vi "task3_BINARY2DEC_CONVERTER.vi"() -> ()   [LabVIEW 2017]
panel:
  out "display":dbl
  in  "2^0":bool
  in  "2^1":bool
  in  "2^2":bool
  in  "2^3":bool
  in  "2^4":bool
  in  "2^5":bool
  in  "2^6":bool
  in  "2^7":bool
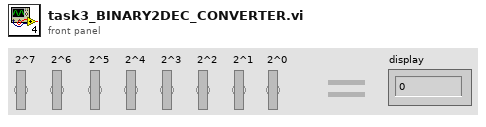
[diagram p1: front panel]
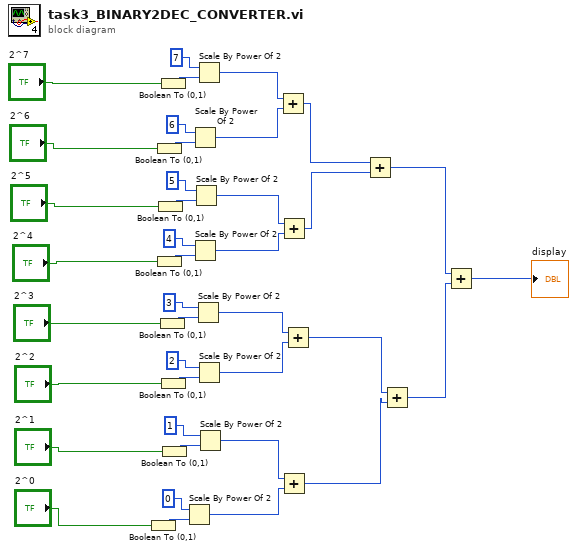
[diagram p0: block diagram]
diagram:
  n1 = Boolean To (0,1)(Boolean="2^0") -> (0, 1=w39:i16)
  n2 = Boolean To (0,1)(Boolean="2^6") -> (0, 1=w33:i16)
  n3 = Boolean To (0,1)(Boolean="2^4") -> (0, 1=w35:i16)
  n4 = Boolean To (0,1)(Boolean="2^5") -> (0, 1=w34:i16)
  n5 = Boolean To (0,1)(Boolean="2^3") -> (0, 1=w36:i16)
  n6 = Boolean To (0,1)(Boolean="2^7") -> (0, 1=w32:i16)
  n7 = Boolean To (0,1)(Boolean="2^2") -> (0, 1=w37:i16)
  n8 = Boolean To (0,1)(Boolean="2^1") -> (0, 1=w38:i16)
  n9 = Scale By Power Of 2(n=0, x=w39) -> (x*2^n=w16:i16)
  n10 = Scale By Power Of 2(n=6, x=w33) -> (x*2^n=w22:i16)
  n11 = Scale By Power Of 2(n=4, x=w35) -> (x*2^n=w20:i16)
  n12 = Scale By Power Of 2(n=5, x=w34) -> (x*2^n=w21:i16)
  n13 = Scale By Power Of 2(n=3, x=w36) -> (x*2^n=w19:i16)
  n14 = Scale By Power Of 2(n=7, x=w32) -> (x*2^n=w23:i16)
  n15 = Scale By Power Of 2(n=2, x=w37) -> (x*2^n=w18:i16)
  n16 = Scale By Power Of 2(n=1, x=w38) -> (x*2^n=w17:i16)
  n17 = Add(x=w23, y=w22) -> (x+y=w12:i16)
  n18 = Add(x=w21, y=w20) -> (x+y=w13:i16)
  n19 = Add(x=w17, y=w16) -> (x+y=w14:i16)
  n20 = Add(x=w19, y=w18) -> (x+y=w15:i16)
  n21 = Add(x=w12, y=w13) -> (x+y=w11:i16)
  n22 = Add(x=w15, y=w14) -> (x+y=w10:i16)
  n23 = Add(x=w11, y=w10) -> (x+y=→"display":i16)
